vi "Read MSG Queue.vi"(8 "error in (no error)":errorcluster, 11 "SEQ in":refnum<class "SEQ.lvclass">) -> (0 "error out":errorcluster, 2 "MSG Queue":refnum<queue>, 3 "SEQ out":refnum<class "SEQ.lvclass">)   [LabVIEW 2016, in "Sequence Composition.lvlib" / "SEQ.lvclass"]
uses:
  SEQ.lvclass
  SEQ.lvclass/SEQ.ctl
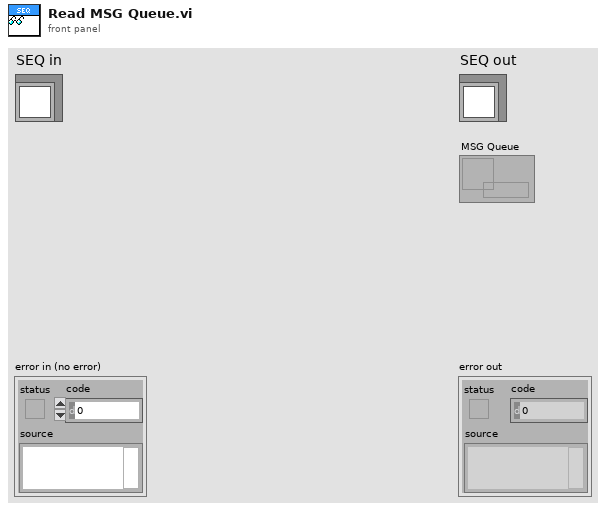
[diagram p1: front panel]
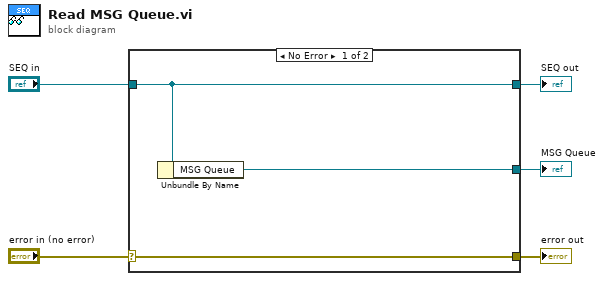
[diagram p0: block diagram]
diagram:
  n1 = case shown="No Error" "error in (no error)" {
    selector: "error in (no error)" -> [w8 w9]
    tunnel: [w8 w9] -> w4
    tunnel: [w7 w10] -> w2
    tunnel: "SEQ in" -> [w7 w10]
    tunnel: [w6 _] -> w1
    frame No Error {
      n2 = Unbundle By Name(w7) -> ("MSG Queue"=w6:refnum<queue>)
    }
    frame Error {
    }
  }
  "error out" <- w4
  "SEQ out" <- w2
  "MSG Queue" <- w1
